vi "TDK-Lambda Z Set and Read Output Parameters.vi"() -> ()   [LabVIEW 2012]
doc: "This example shows how to set and take readings.\n\n<b>Note:</b>\n1. Set Property Communication Parameters\n2. Set Required Output Values and then RUN\n\nNote:\nSet OVP value above 5V and at least 5% higher then Voltage Limit"
uses:
  TDK-Lambda Z.lvlib
panel:
  in  "Configuration":T1={"Address"=6, "Baud Rate"=9600, "Language Selector"=1} {"Language Selector" items=["GEN", "SCPI"]; "Baud Rate" items=["1200"=1200, "2400"=2400, "4800"=4800, "9600"=9600, "19200"=19200, "38400"=38400, "57600"=57600, "115200"=115200]}
  in  "OVP (0V)":dbl format="%.4f"
  in  "UV Level (0V)":dbl format="%.4f"
  in  "Current Limit (0A)":dbl format="%.4f"
  in  "Voltage Limit (0V)":dbl format="%.4f"
  out "Output Current":dbl format="%.4f"
  out "Output Voltage (V)":dbl format="%.4f"
  in  "Output (F: Off)":bool
  in  "ID Query (True)":bool
  in  "Reset(True)":bool
  in  "VISA resource name":refnum<visa-resource-name>
  # "(c) 2014-2015 TDK-Lambda.  ALL RIGHTS RESERVED."
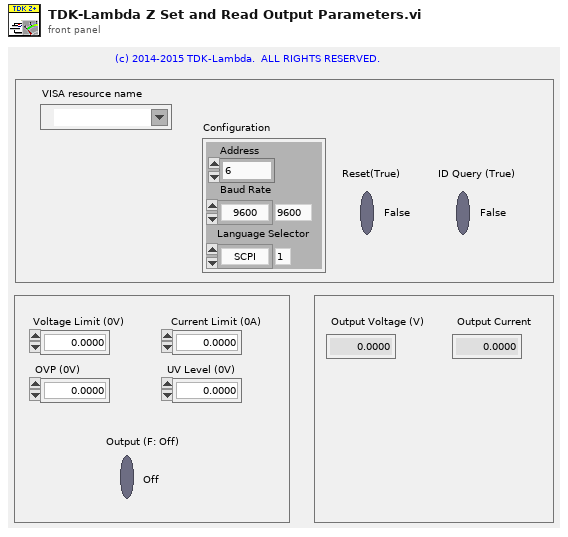
[diagram p1: front panel]
types:
  T1 = cluster{"Address":i16, "Baud Rate":u32, "Language Selector":i16}
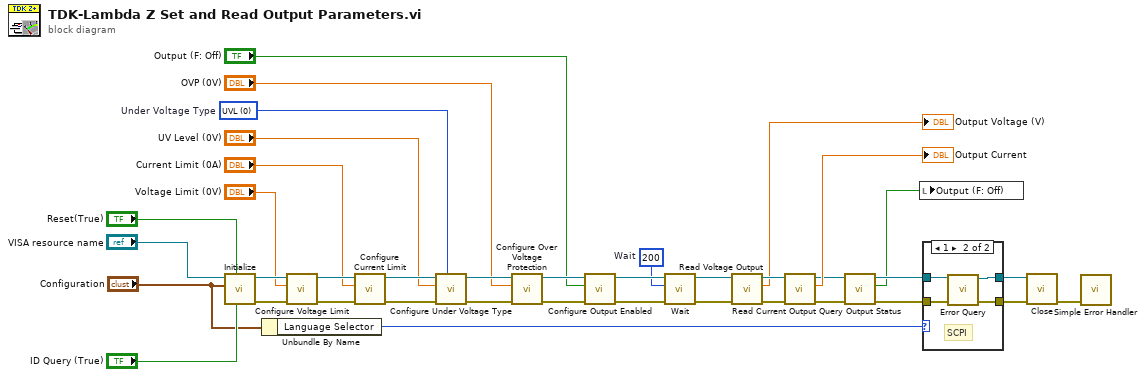
[diagram p0: block diagram]
diagram:
  w7 = u32 200  # Wait
  w8 = u16 0 items=["UVL", "UVP"]  # Under Voltage Type
  n1 = call "Initialize.vi"("ID Query (True)"="ID Query (True)", "Reset(True)"="Reset(True)", "Configuration"="Configuration", "VISA resource name"="VISA resource name") -> ("error out"=w20:errorcluster, "VISA resource name out"=w19:refnum<visa-resource-name>)  [unwired: 6 in]
  n2 = Unbundle By Name("Configuration") -> ("Language Selector"=w21:i16)
  n3 = call "Configure Voltage Limit.vi"("error in (no error)"=w20, "Voltage Limit (0V)"="Voltage Limit (0V)", "VISA resource name"=w19) -> ("error out"=w31:errorcluster, "VISA resource name out"=w38:refnum<visa-resource-name>)  [unwired: 7 in]
  n4 = call "Configure Current Limit.vi"("error in (no error)"=w31, "Current Limit (0A)"="Current Limit (0A)", "VISA resource name"=w38) -> ("error out"=w30:errorcluster, "VISA resource name out"=w37:refnum<visa-resource-name>)  [unwired: 7 in]
  n5 = call "Configure Under Voltage Type.vi"("Under Voltage Type  (0: UVL)"=w8, "error in (no error)"=w30, "UV Level (0V)"="UV Level (0V)", "VISA resource name"=w37) -> ("error out"=w29:errorcluster, "VISA resource name out"=w36:refnum<visa-resource-name>)  [unwired: 6 in]
  n6 = call "Configure Over Voltage Protection.vi"("error in (no error)"=w29, "OVP (0V)"="OVP (0V)", "VISA resource name"=w36) -> ("error out"=w28:errorcluster, "VISA resource name out"=w35:refnum<visa-resource-name>)  [unwired: 7 in]
  n7 = call "Configure Output Enabled.vi"("error in (no error)"=w28, "Enable Output (F: Off)"="Output (F: Off)", "VISA resource name"=w35) -> ("error out"=w27:errorcluster, "VISA resource name out"=w34:refnum<visa-resource-name>)  [unwired: 7 in]
  n8 = call "Wait.vi"("error in (no error)"=w27, "Wait (1mS)"=w7, "VISA resource name"=w34) -> ("error out"=w26:errorcluster, "VISA resource name out"=w33:refnum<visa-resource-name>)  [unwired: 7 in]
  n9 = call "Read Voltage Output .vi"("error in (no error)"=w26, "VISA resource name"=w33) -> ("error out"=w25:errorcluster, "Output Voltage (V)"=→"Output Voltage (V)":dbl, "VISA resource name out"=w32:refnum<visa-resource-name>)  [unwired: 7 in]
  n10 = call "Read Current Output.vi"("error in (no error)"=w25, "VISA resource name"=w32) -> ("error out"=w4:errorcluster, "Output Current (A)"=→"Output Current":dbl, "VISA resource name out"=w5:refnum<visa-resource-name>)  [unwired: 7 in]
  n11 = call "Query Output Status.vi"("error in (no error)"=w4, "VISA resource name"=w5) -> ("error out"=w2:errorcluster, "Output On"=w1:bool, "VISA resource name out"=w3:refnum<visa-resource-name>)  [unwired: 7 in]
  n12 = local write "Output (F: Off)"(w1) -> ()
  n13 = case shown="1" w21 {
    tunnel: w3 -> [w40 w44]
    tunnel: w2 -> [w39 w43]
    tunnel: [w40 w42] -> w23
    tunnel: [w39 w41] -> w22
    frame 0, Default {
      # "GEN"
    }
    frame 1 {
      # "SCPI"
      n14 = call "Error Query.vi"("error in (no error)"=w43, "VISA resource name"=w44) -> ("error out"=w41:errorcluster, "VISA resource name out"=w42:refnum<visa-resource-name>)  [unwired: 6 in, 2 out]
    }
  }
  n15 = call "Close.vi"("error in (no error)"=w22, "VISA resource name"=w23) -> ("error out"=w18:errorcluster)  [unwired: 9 in]
  n16 = call <vilib>:"Simple Error Handler.vi"("error in (no error)"=w18) -> ()  [unwired: 4 in, 5 out]
